vi "Configure Channel.vi"(8 "error in (no error)":errorcluster, 10 "Settings":T1 {"Fall Time" format="%#_g s"; "Rise Time" format="%#_g s"; "Pulse Width" format="%#_g s"; "Symmetry" format="%#_g %"; "Phase" format="%#_g °"; "Offset" format="%#_g V"; "Amplitude" format="%#_g V"; "Frequency" format="%#_g Hz"}, 11 "FunctionGenerator in":refnum<class "FunctionGenerator.lvclass">) -> (0 "error out":errorcluster, 3 "FunctionGenerator out":refnum<class "FunctionGenerator.lvclass">)   [LabVIEW 2019, in "FunctionGenerator.lvlib" / "FunctionGenerator.lvclass"]
uses:
  Library/FunctionGenerator.lvclass
  C:/Users/Public/Documents/Development/builds/Instruments/Instruments.lvlibp/Library/Instruments.lvclass
  Custom Controls/WaveformSettings.ctl
  Custom Controls/WaveformMode.ctl
  Library/FunctionGenerator.lvclass/FunctionGenerator.ctl
  builds/Instruments/Instruments.lvlibp/Private/Polymorphic/Special/Event from String.vi
  builds/Instruments/Instruments.lvlibp/Accessors/Command with Logging.vi
  builds/Instruments/Instruments.lvlibp/Library/Instruments.lvclass
  builds/Engine/Engine.lvlibp/Project/Engine.lvclass
  builds/Instruments/Instruments.lvlibp
  C:/Users/Public/Documents/Development/builds/Engine/Engine.lvlibp/Project/Engine.lvclass
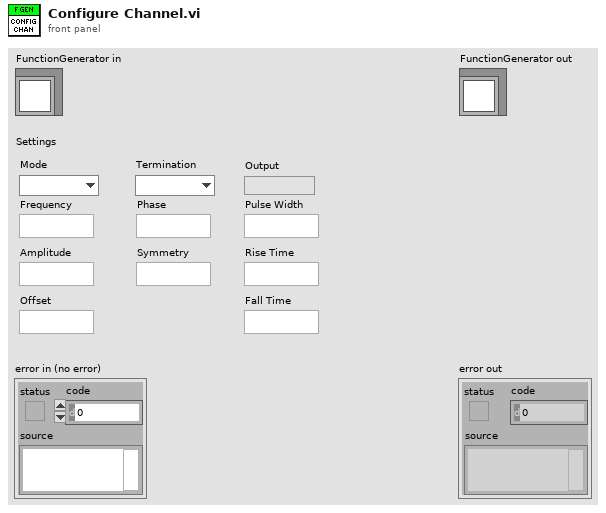
[diagram p1: front panel]
types:
  T1 = typedef "FunctionGenerator.lvlib/FunctionGenerator.lvclass/WaveformSettings.ctl" = cluster{"Frequency":dbl, "Amplitude":dbl, "Offset":dbl, "Phase":dbl, "Symmetry":dbl, "Pulse Width":dbl, "Rise Time":dbl, "Fall Time":dbl, "Mode":T2, "Termination":enum16{"50_Ohm", "High_Z"}, "Output":bool}
  T2 = typedef "FunctionGenerator.lvlib/FunctionGenerator.lvclass/WaveformMode.ctl" = enum16{"Sine", "Square", "Ramp", "Pulse", "Arbitrary", "Triangle", "Noise", "DC"}
  T3 = cluster{"Timestamp":timestamp, "Description":string, "Data":string}
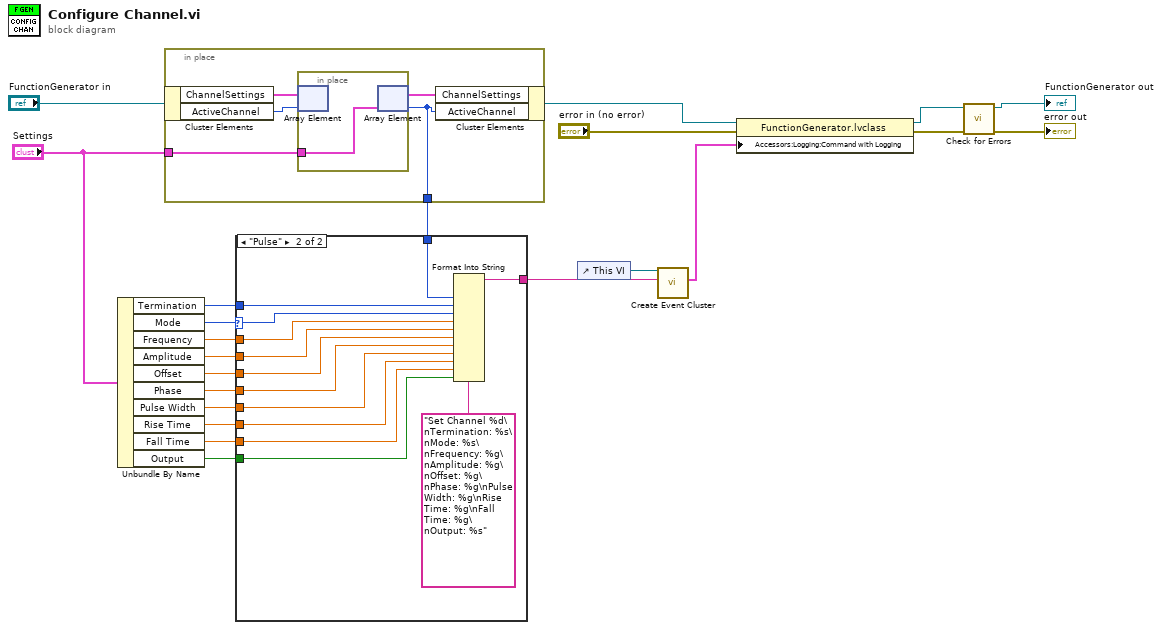
[diagram p0: block diagram]
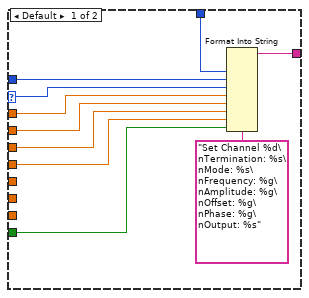
[diagram p2: hidden frame]
diagram:
  n1 = Unbundle By Name("Settings") -> ("Termination"=w18:enum16{"50_Ohm", "High_Z"}, "Mode"=w4:T2, "Frequency"=w9:dbl, "Amplitude"=w8:dbl, "Offset"=w7:dbl, "Phase"=w6:dbl, "Pulse Width"=w3:dbl, "Rise Time"=w2:dbl, "Fall Time"=w1:dbl, "Output"=w5:bool)
  n2 = in-place {
    in-place-border: "Settings" -> [w25]
    in-place-border: [w23] -> w19
    n3 = in-place-cluster #1("FunctionGenerator in") -> ("ChannelSettings"=w27:T1[], "ActiveChannel"=w24:i32)
    n4 = in-place {
      in-place-border: w25 -> [w28]
      n5 = in-place-array #2(w27, w24) -> ()  [unwired: 1 out]
      n6 = in-place-array #2(w28) -> (w26:T1[], w23:i32)
    }
    n7 = in-place-cluster #1("ChannelSettings"=w26, "ActiveChannel"=w23) -> (w21:refnum<class "FunctionGenerator.lvclass">)
  }
  n8 = case shown="\"Pulse\"" w4 {
    selector: w4 -> [w29 w43]
    tunnel: w19 -> [w37 w50]
    tunnel: w18 -> [w36 w49]
    tunnel: [w35 w48] -> w14
    tunnel: w9 -> [w34 w47]
    tunnel: w8 -> [w33 w46]
    tunnel: w7 -> [w32 w45]
    tunnel: w6 -> [w31 w44]
    tunnel: w5 -> [w30 w42]
    tunnel: w3 -> [_ w39]
    tunnel: w2 -> [_ w40]
    tunnel: w1 -> [_ w41]
    frame Default {
      n9 = Format Into String(format string="Set Channel %d\nTermination: %s\nMode: %s\nFrequency: %g\nAmplitude: %g\nOffset: %g\nPhase: %g\nOutput: %s", w37, w36, w29, w34, w33, w32, w31, w30) -> (resulting string=w35:string)  [unwired: 2 in, 1 out]
    }
    frame "Pulse" {
      n10 = Format Into String(format string="Set Channel %d\nTermination: %s\nMode: %s\nFrequency: %g\nAmplitude: %g\nOffset: %g\nPhase: %g\nPulse Width: %g\nRise Time: %g\nFall Time: %g\nOutput: %s", w50, w49, w43, w47, w46, w45, w44, w39, w40, w41, w42) -> (resulting string=w48:string)  [unwired: 2 in, 1 out]
    }
  }
  n11 = control-ref of="This VI"() -> (w15:refnum<vi>)
  n12 = call-poly "Create Event Cluster.vi"("Value"=w14, "VI Refnum"=w15) -> ("Event Data"=w13:T3)  [unwired: 9 in]
  n13 = property class="FunctionGenerator.lvclass"(reference=w21, error in="error in (no error)", "Accessors:Logging:Command with Logging"=w13) -> (reference out=w11:refnum<class "FunctionGenerator.lvclass">, error out=w16:errorcluster)
  n14 = call "Check for Errors.vi"("error in"=w16, "Engine in"=w11) -> ("error out"=→"error out":errorcluster, "Engine out"=→"FunctionGenerator out":refnum<class "FunctionGenerator.lvclass">)  [unwired: 8 in]
